vi "Mercury_GCS_Simple_Test.vi"() -> ()   [LabVIEW 2011]
doc: "This simple test VI is a stand-alone sample application. Use the \nHelp?Show Context Help menu sequence in the LabVIEW environment to display the Context Help window with the VI and control/indicator descriptions.\nSpecify \n¢ System number (= 1 in a one-system configuration),\n¢ Interface (RS232, RS232 DaisyChain, USB or USB DaisyChain),\n¢ For Interface = RS232 or RS232 DaisyChain: appropriate port number and RS232 baud rate, or\n¢ For Interface = USB or USB DaisyChain: appropriate Serial Number of the controller to connect to or if you want to search for the controller, and\n¢ For Interface = RS232 DaisyChain or USB DaisyChain: select if you want to register the DaisyChain if it is not already open only (FALSE) or in any case (TRUE), if you want to call a dialog to select the connected Mercury controller from a list (TRUE) or if you know the Device ID of the controller to connect (FALSE, Device ID must match the device ID of the controller in the DaisyChain network). If one device of a DaisyChain is already connected with LabVIEW, do not switch Register DC to TRUE; and\n¢ Timeout value (in milliseconds).\nThen start the VI. The VI will open the chosen communication port and query for the identification string of the connected Mercury controller. The diagram shows how to combine the driver and support VIs for these tasks."
panel:
  in  "DaisyChain settings":T1={"Register DC"=FALSE, "DaisyChain Search?"=TRUE, "Device ID"=1}
  in  "USB settings":cluster{"S/N":string, "USB Search?":bool}={"S/N"="", "USB Search?"=TRUE}
  in  "RS232 settings":cluster{"Portnumber":i32, "Baudrate":u16}={"Portnumber"=0, "Baudrate"=3} {"Portnumber" items=["COM1", "COM2", "COM3", "COM4", "COM5", "COM6", "COM7", "COM8", "COM9", "COM10", "COM11", "COM12", "COM13", "COM14", "COM15", "COM16", "COM17", "COM18", "COM19", "COM20", "COM21", "COM22", "COM23", "COM24", "COM25", "COM26", "COM27", "COM28", "COM29", "COM30"]; "Baudrate" items=["9600", "14400", "19200", "38400", "57600", "115200"]}
  in  "Interface":u16(ring) items=["RS232", "RS232 DaisyChain", "USB", "USB_DaisyChain"]
  in  "System no.":i32=1 min=1 step=1
  in  "error in":errorcluster
  in  "Timeout":u32=5000
  out "error out":errorcluster
  out "Identification":string
  # "Simple Mercury GCS Communication \nTest Program"
  # "Select Interface settings first, then start the VI. The VI will open the chosen \ncommunication port and query for the identification string (*IDN?) of the connected Mercury controller\nwith GCS firmware. See VI and control/indicator information for details."
  # "Only for\nInterface = \nRS232 or\nRS232\nDaisyChain:"
  # "Only for\nInterface = \nUSB or USB DaisyChain"
  # "Only for \nInterface =\nRS232/USB \nDaisyChain:"
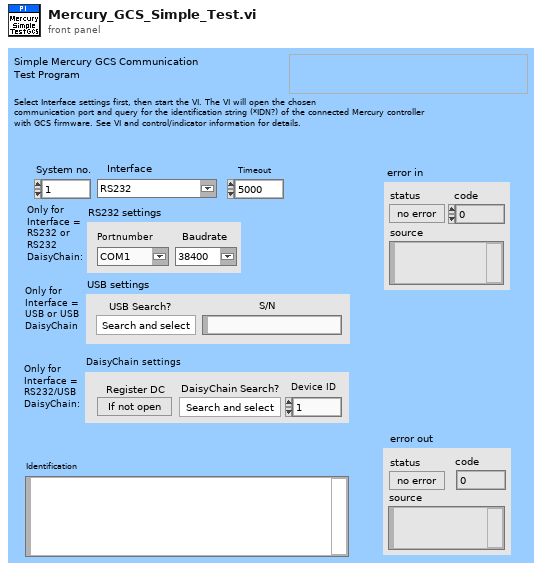
[diagram p1: front panel]
types:
  T1 = cluster{"Register DC":bool, "DaisyChain Search?":bool, "Device ID":i32}
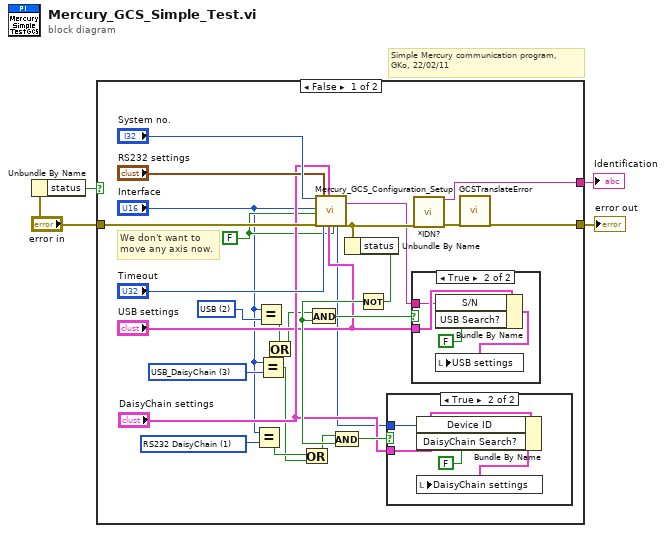
[diagram p0: block diagram]
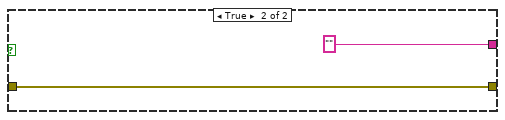
[diagram p4: hidden frame]
diagram:
  # "Simple Mercury communication program,\nGKo, 22/02/11"
  n1 = Unbundle By Name("error in") -> ("status"=w1:bool)
  n2 = case shown="False" w1 {
    tunnel: [w30 "" ("Identification")] -> w4
    tunnel: [w29 w39] -> w3
    tunnel: "error in" -> [w26 w39]
    frame False {
      w7 = u16 1 items=["RS232", "RS232 DaisyChain", "USB", "USB_DaisyChain"] ("Interface")
      w13 = u16 2 items=["RS232", "RS232 DaisyChain", "USB", "USB_DaisyChain"] ("Interface")
      w12 = u16 3 items=["RS232", "RS232 DaisyChain", "USB", "USB_DaisyChain"] ("Interface")
      w15 = FALSE ("Can axis be moved?")
      # "We don't want to\nmove any axis now."
      n3 = Equal?(x="Interface", y=w7) -> (x = y?=w10:bool)
      n4 = Equal?(x="Interface", y=w13) -> (x = y?=w14:bool)
      n5 = Equal?(x="Interface", y=w12) -> (x = y?=w6:bool)
      n6 = Or(x=w14, y=w6) -> (x .or. y?=w11:bool)
      n7 = Or(x=w10, y=w6) -> (x .or. y?=w8:bool)
      n8 = call "Mercury_GCS_Configuration_Setup.vi"("System no."="System no.", "Interface"="Interface", "All axes?"=w15, "error in"=w26, "RS232 settings"="RS232 settings", "Timeout"="Timeout", "DaisyChain settings"="DaisyChain settings", "USB settings"="USB settings", "Switch servo on?"=w15) -> ("Device ID out"=w16:i32, "SN out"=w5:string, "error out"=w23:errorcluster)  [unwired: 4 in, 4 out]
      n9 = Unbundle By Name(w23) -> ("status"=w22:bool)
      n10 = Not(x=w22) -> (.not. x?=w20:bool)
      n11 = And(x=w11, y=w20) -> (x .and. y?=w21:bool)
      n12 = And(x=w8, y=w20) -> (x .and. y?=w19:bool)
      n13 = case shown="True" w19 {
        tunnel: "DaisyChain settings" -> [_ w34]
        tunnel: w16 -> [_ w33]
        frame False {
        }
        frame True {
          n14 = Bundle By Name(cluster=w34, "Device ID"=w33, "DaisyChain Search?"=FALSE ("USB Search?")) -> (w31:T1)
          n15 = local write "DaisyChain settings"(w31) -> ()
        }
      }
      n16 = case shown="True" w21 {
        tunnel: "USB settings" -> [_ w38]
        tunnel: w5 -> [_ w37]
        frame False {
        }
        frame True {
          n17 = Bundle By Name(cluster=w38, "S/N"=w37, "USB Search?"=FALSE) -> (w35:cluster{"S/N":string, "USB Search?":bool})
          n18 = local write "USB settings"(w35) -> ()
        }
      }
      n19 = call "*IDN?.vi"("error in"=w23) -> ("Identification"=w30:string, "error out"=w28:errorcluster)  [unwired: 17 in]
      n20 = call "GCSTranslateError.vi"("error in"=w28) -> ("error out"=w29:errorcluster)  [unwired: 16 in, 2 out]
    }
    frame True {
    }
  }
  "Identification" <- w4
  "error out" <- w3
